vi "GetHistory.vi"(8 "Error Input":errorcluster, 10 "SessionId":string, 11 "LiteAgentSDK Input":refnum<k24>) -> (0 "Error Output":errorcluster, 2 "HistoryJson":string, 3 "LiteAgentSDK Output":refnum<k24>)   [LabVIEW 2017, in "LiteAgentSDK.lvlib"]
uses:
  LiteAgentSDK.lvlib
  C:/Users/Jan/Projects/LiteAgentSDK-LabVIEW/Source/Bin/LiteAgentSDK.LabVIEW.dll
  Bin/LiteAgentSDK.LabVIEW.dll
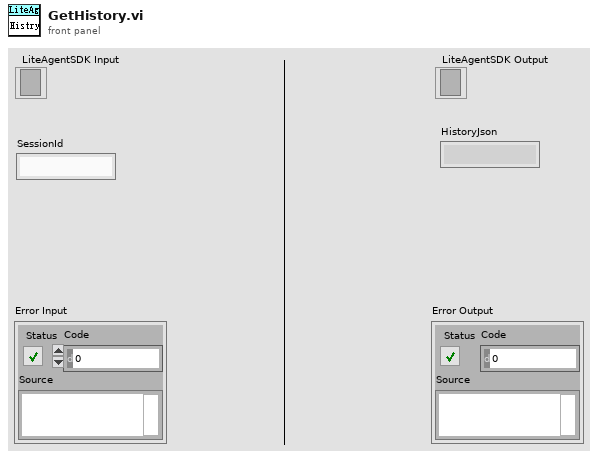
[diagram p1: front panel]
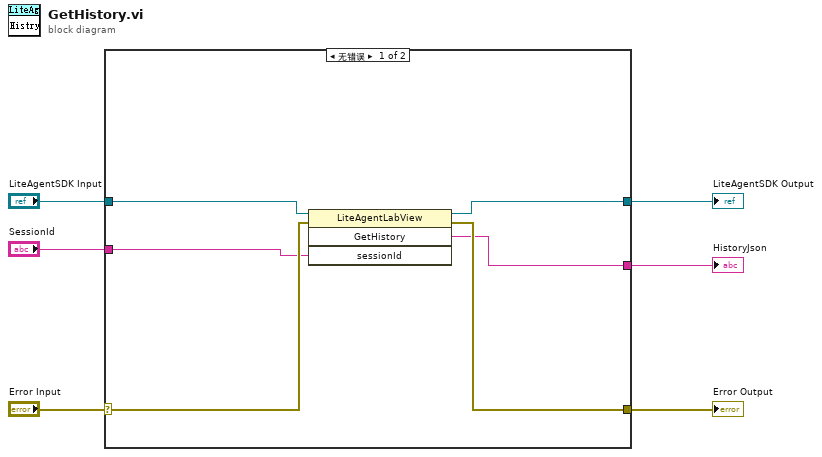
[diagram p0: block diagram]
diagram:
  n1 = case shown="无错误" "Error Input" {
    selector: "Error Input" -> [w11 w13]
    tunnel: "LiteAgentSDK Input" -> [w12 w14]
    tunnel: [w9 w14] -> w1
    tunnel: [w10 w13] -> w5
    tunnel: "SessionId" -> [w8 _]
    tunnel: [w7 _] -> w3
    frame No Error {
      n2 = invoke on="调用节点" class="LiteAgentLabView" method="GetHistory"(reference=w12, error in=w11, "sessionId"=w8) -> (reference out=w9:refnum<k24>, error out=w10:errorcluster, "GetHistory"=w7:string)  [unwired: 1 in, 1 out]
    }
    frame Error {
    }
  }
  "Error Output" <- w5
  "HistoryJson" <- w3
  "LiteAgentSDK Output" <- w1
